vi "Start Async.vi"(8 "error in (no error)":errorcluster, 11 "gRPC Server in":refnum<class "PluginCore.lvclass">) -> (0 "error out":errorcluster, 3 "gRPC Server out":refnum<class "PluginCore.lvclass">)   [LabVIEW 2021, in "CIFCorePlugin_server.lvlib" / "PluginCore.lvclass"]
uses:
  PluginCore.lvclass
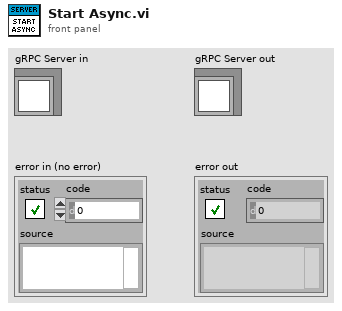
[diagram p1: front panel]
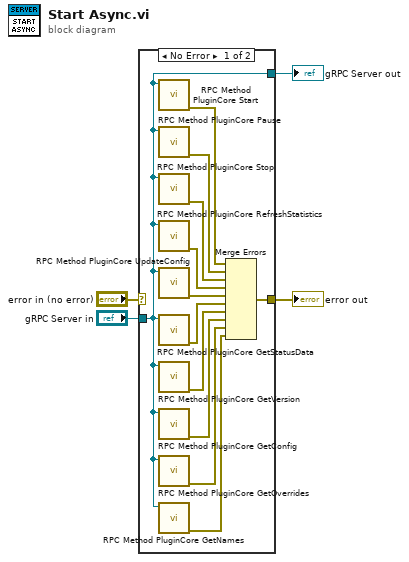
[diagram p0: block diagram]
diagram:
  n1 = case shown="No Error" "error in (no error)" {
    selector: "error in (no error)" -> [_ w18]
    tunnel: [w16 w18] -> w3
    tunnel: [w15 w17] -> w1
    tunnel: "gRPC Server in" -> [w15 w17]
    frame No Error {
      n2 = call "RPC Method PluginCore Start.vi"("OOP Server in"=w15) -> ("error out"=w14:errorcluster)  [unwired: 9 in, 1 out]
      n3 = call "RPC Method PluginCore Pause.vi"("OOP Server in"=w15) -> ("error out"=w13:errorcluster)  [unwired: 9 in, 1 out]
      n4 = call "RPC Method PluginCore Stop.vi"("OOP Server in"=w15) -> ("error out"=w12:errorcluster)  [unwired: 9 in, 1 out]
      n5 = call "RPC Method PluginCore RefreshStatistics.vi"("OOP Server in"=w15) -> ("error out"=w11:errorcluster)  [unwired: 9 in, 1 out]
      n6 = call "RPC Method PluginCore UpdateConfig.vi"("OOP Server in"=w15) -> ("error out"=w10:errorcluster)  [unwired: 9 in, 1 out]
      n7 = call "RPC Method PluginCore GetStatusData.vi"("OOP Server in"=w15) -> ("error out"=w9:errorcluster)  [unwired: 9 in, 1 out]
      n8 = call "RPC Method PluginCore GetVersion.vi"("OOP Server in"=w15) -> ("error out"=w8:errorcluster)  [unwired: 9 in, 1 out]
      n9 = call "RPC Method PluginCore GetConfig.vi"("OOP Server in"=w15) -> ("error out"=w7:errorcluster)  [unwired: 9 in, 1 out]
      n10 = call "RPC Method PluginCore GetOverrides.vi"("OOP Server in"=w15) -> ("error out"=w6:errorcluster)  [unwired: 9 in, 1 out]
      n11 = call "RPC Method PluginCore GetNames.vi"("OOP Server in"=w15) -> ("error out"=w5:errorcluster)  [unwired: 9 in, 1 out]
      n12 = Merge Errors(w14, w13, w12, w11, w10, w9, w8, w7, w6, w5) -> (w16:errorcluster)
    }
    frame Error {
    }
  }
  "error out" <- w3
  "gRPC Server out" <- w1
